vi "testVi.vi"(8 "error in (no error)":errorcluster, 10 "Numeric":i32, 11 "TestClass in":refnum<class "TestClass.lvclass">) -> (0 "error out":errorcluster, 2 "x+1":i32, 3 "TestClass out":refnum<class "TestClass.lvclass">)   [LabVIEW 2015, in "TestClass.lvclass"]
uses:
  TestClass.lvclass
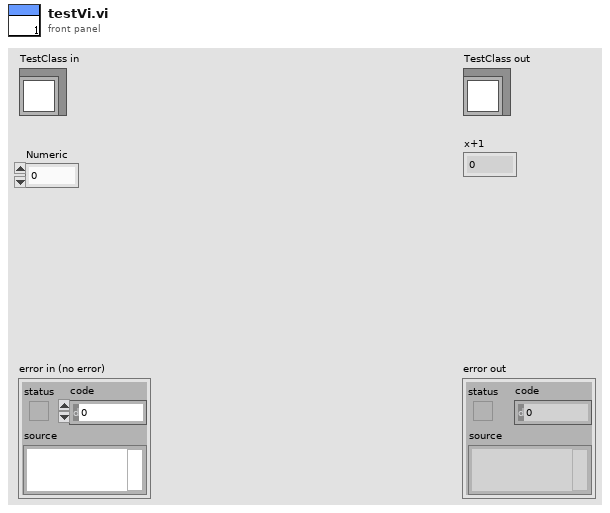
[diagram p1: front panel]
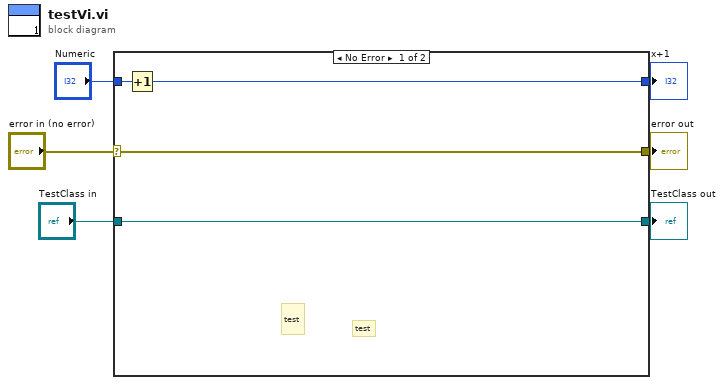
[diagram p0: block diagram]
diagram:
  n1 = case shown="No Error" "error in (no error)" {
    selector: "error in (no error)" -> [w9 w12]
    tunnel: [w9 w12] -> w5
    tunnel: [w10 w11] -> w3
    tunnel: "TestClass in" -> [w10 w11]
    tunnel: "Numeric" -> [w8 _]
    tunnel: [w7 _] -> w1
    frame No Error {
      # "test"
      # "test"
      n2 = Increment(x=w8) -> (x+1=w7:i32)
    }
    frame Error {
    }
  }
  "error out" <- w5
  "TestClass out" <- w3
  "x+1" <- w1
